vi "makeCall.vi"(8 "error in (no error)":errorcluster, 10 "call":u8, 11 "BingoBoard in":refnum<class "BingoBoard.lvclass">) -> (0 "error out":errorcluster, 2 "won?":bool, 3 "BingoBoard out":refnum<class "BingoBoard.lvclass">)   [LabVIEW 2017, in "BingoBoard.lvclass"]
uses:
  BingoBoard.lvclass
  BoardField/BoardField.lvclass
  BingoBoard.lvclass/BingoBoard.ctl
  BoardField/BoardField.lvclass/BoardField.ctl
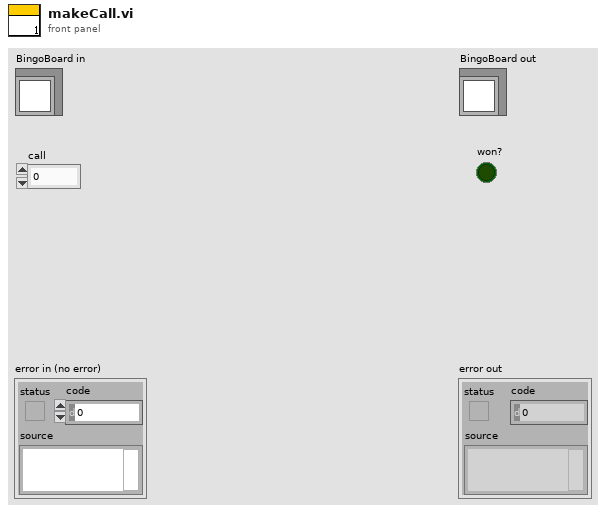
[diagram p1: front panel]
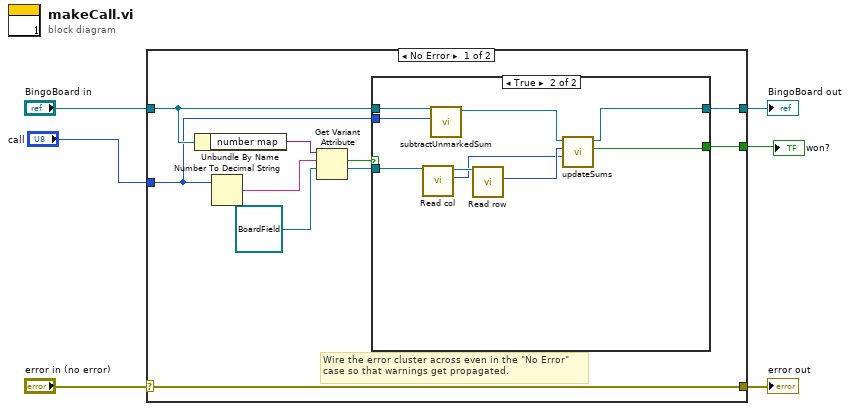
[diagram p0: block diagram]
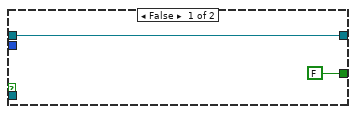
[diagram p2: hidden frame]
diagram:
  n1 = case shown="No Error" "error in (no error)" {
    selector: "error in (no error)" -> [w16 w29]
    tunnel: [w16 w29] -> w5
    tunnel: [w11 w28] -> w3
    tunnel: "BingoBoard in" -> [w10 w28]
    tunnel: "call" -> [w7 _]
    tunnel: [w9 _] -> w1
    frame No Error {
      # "Wire the error cluster across even in the \"No Error\"\ncase so that warnings get propagated."
      n2 = Unbundle By Name(w10) -> ("number map"=w15:variant)
      n3 = Number To Decimal String(number=w7) -> (decimal integer string=w14:string)  [unwired: 1 in]
      n4 = Get Variant Attribute(Variant=w15, name=w14, default value (empty Variant)=refnum<class "BoardField.lvclass"> refnum ("field")) -> (found=w12:bool, value=w8:refnum<class "BoardField.lvclass">)  [unwired: 1 in, 2 out]
      n5 = case shown="True" w12 {
        tunnel: [w18 w20] -> w11
        tunnel: w10 -> [w18 w25]
        tunnel: [FALSE ("won?") w19] -> w9
        tunnel: w8 -> [_ w27]
        tunnel: w7 -> [_ w24]
        frame False {
        }
        frame True {
          n6 = call "Read col.vi"("BoardField in"=w27) -> ("col"=w21:u8, "BoardField out"=w26:refnum<class "BoardField.lvclass">)  [unwired: 8 in, 1 out]
          n7 = call "subtractUnmarkedSum.vi"("Numeric"=w24, "BingoBoard in"=w25) -> ("output cluster"=w23:refnum<class "BingoBoard.lvclass">)  [unwired: 9 in]
          n8 = call "Read row.vi"("BoardField in"=w26) -> ("row"=w22:u8)  [unwired: 8 in, 2 out]
          n9 = call-dynamic "updateSums.vi"("col"=w21, "row"=w22, "BingoBoard in"=w23) -> ("won?"=w19:bool, "BingoBoard out"=w20:refnum<class "BingoBoard.lvclass">)  [unwired: 6 in, 1 out]
        }
      }
    }
    frame Error {
    }
  }
  "error out" <- w5
  "BingoBoard out" <- w3
  "won?" <- w1
